vi "Global AMS.vi"() -> ()   [LabVIEW 2013]
uses:
  Connection Information Cluster.ctl
  DB - Logon Info.ctl
  DB - Logon Extra Info.ctl
panel:
  out "DB Available":bool
  in  "Server MasterData\\JPG Folder":path=path "c:/temp/SRTRS4070/MasterData/JPG"
  in  "AMS Connection Information":T1={"Connection "="SQL Server 32bit HPEnvy", "Username"="admin", "Password"="admin123"}
  in  "CMS Connection Information":T1={"Connection "="SQL Server 32bit HPEnvy", "Username"="admin", "Password"="admin123"}
  out "Enable Central Monitoring":bool
  in  "Main Application Directory":path
  out "Temperature Units":string
  in  "Timeout for MessageQ (ms)":i32=1000
  out "MessageQ":refnum<queue>
  in  "DB - Message":bool=TRUE
  in  "[TransactionRunNo]":string
  in  "Minimum Severity Level to Send Out":i32
  in  "[TransactionNo]":string
  in  "NULL TimeStamp":timestamp=timestamp(31593600 s since 1904-01-01)
  out "Logon Extra":T2
  out "Logon":T3={"PlantID"="", "SystemID"="", "UserID"="", "DomainID"="", "LanguageID"="EN", "StationID"=""}
  in  "Date Format":string="%Y-%m-%d"
  in  "Connection Information":T1={"Connection "="SQL Server 32bit HPEnvy", "Username"="admin", "Password"="admin123"}
  out "DB Error":errorcluster
  in  "Date Time Format":string="%Y-%m-%d %H:%M:%S"
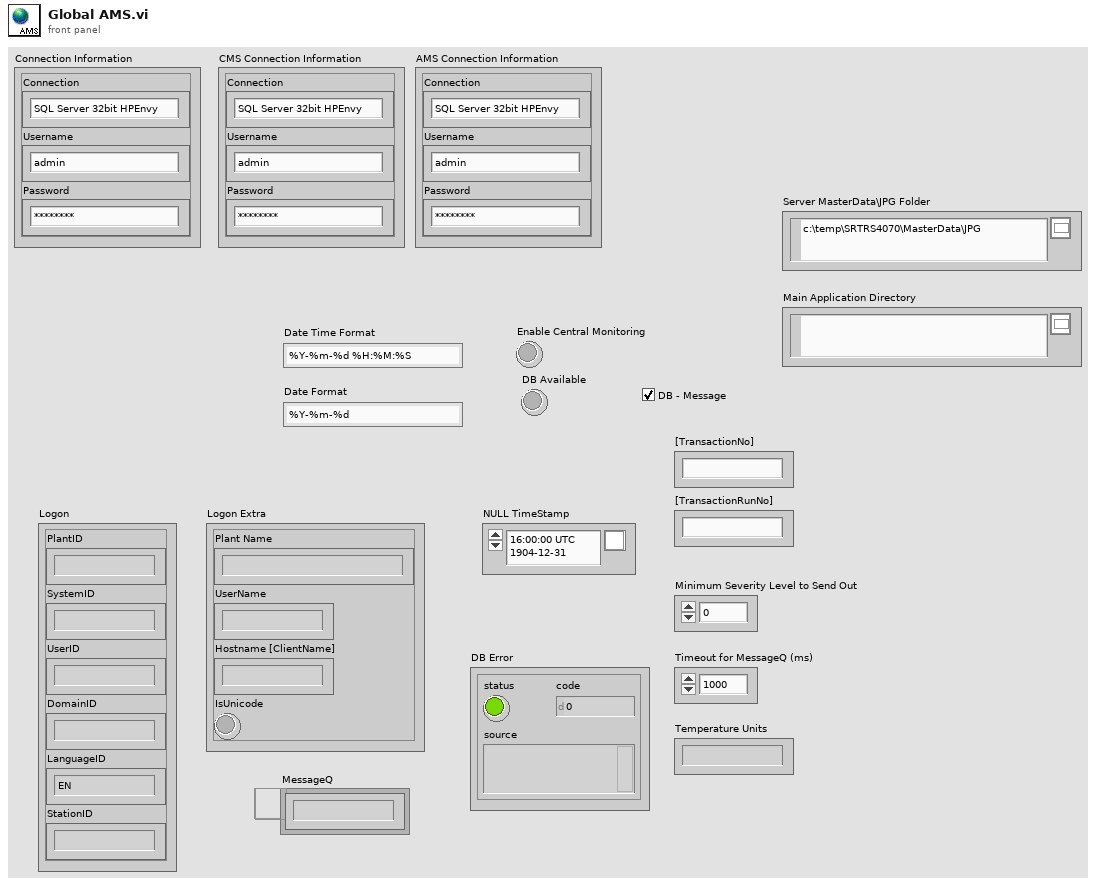
[diagram p1: front panel]
types:
  T1 = typedef "Connection Information Cluster.ctl" = cluster{"Connection ":string, "Username":string, "Password":string}
  T2 = typedef "DB - Logon Extra Info.ctl" = cluster{"Plant Name":string, "UserName":string, "Hostname [ClientName]":string, "IsUnicode":bool}
  T3 = typedef "DB - Logon Info.ctl" = cluster{"PlantID":string, "SystemID":string, "UserID":string, "DomainID":string, "LanguageID":string, "StationID":string}
diagram:
